vi "Word_Set_Bullet_Numbering.vi"(0 "Word._Document":refnum<k7>, 5 "start at":i32, 7 "range start":i32, 9 "range end":i32, 11 "error in (no error)":errorcluster, 12 "list index":i32, 13 "list type":i32(ring)=1 items=["wdBulletGallery"=1, "wdNumberGallery"=2, "wdOutlineNumberGallery"=3]) -> (15 "error out":errorcluster)   [LabVIEW 2017, in "NI_ReportGenerationToolkit.lvlib"]
uses:
  <vilib>/addons/_office/NI_ReportGenerationToolkit.lvlib
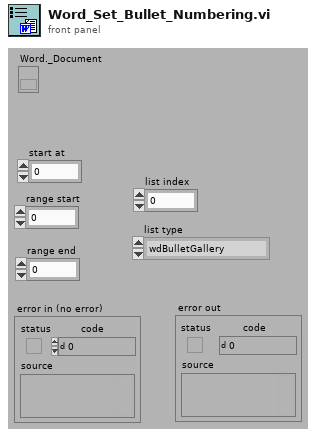
[diagram p1: front panel]
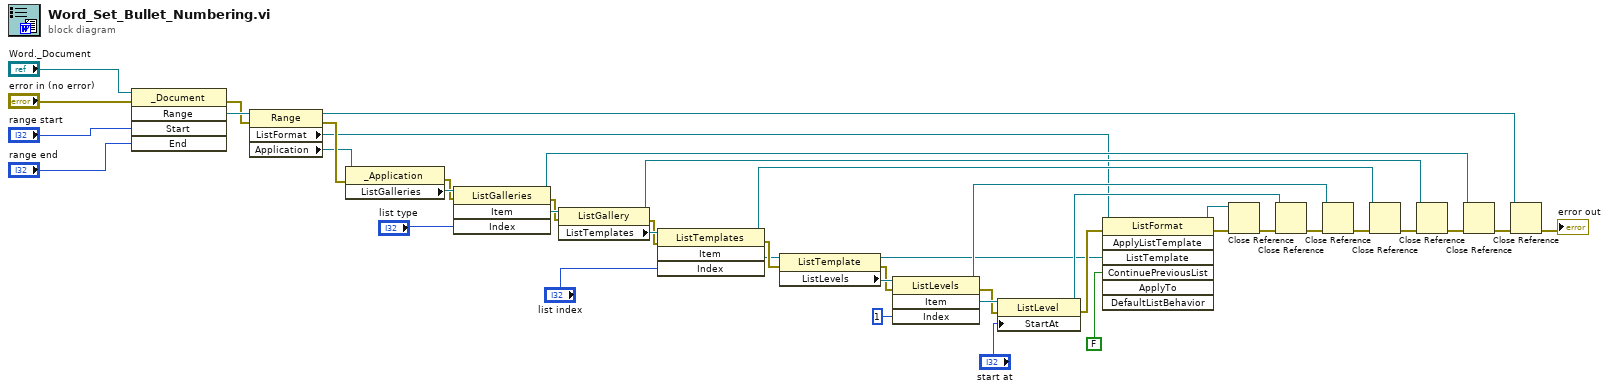
[diagram p0: block diagram]
diagram:
  n1 = invoke class="_Document" method="Range"(reference="Word._Document", error in="error in (no error)", "Start"="range start", "End"="range end") -> (error out=w26:errorcluster, "Range"=w36:refnum<k7>)  [unwired: 1 in, 3 out]
  n2 = property class="Range"(reference=w36, error in=w26) -> (reference out=w14:refnum<k7>, error out=w25:errorcluster, "ListFormat"=w4:refnum<k7>, "Application"=w7:refnum<k7>)
  n3 = property class="_Application"(reference=w7, error in=w25) -> (error out=w32:errorcluster, "ListGalleries"=w37:refnum<k7>)  [unwired: 1 out]
  n4 = invoke class="ListGalleries" method="Item"(reference=w37, error in=w32, "Index"="list type") -> (reference out=w15:refnum<k7>, error out=w31:errorcluster, "Item"=w38:refnum<k7>)  [unwired: 1 in, 1 out]
  n5 = property class="ListGallery"(reference=w38, error in=w31) -> (reference out=w18:refnum<k7>, error out=w30:errorcluster, "ListTemplates"=w39:refnum<k7>)
  n6 = invoke class="ListTemplates" method="Item"(reference=w39, error in=w30, "Index"="list index") -> (reference out=w19:refnum<k7>, error out=w29:errorcluster, "Item"=w9:refnum<k7>)  [unwired: 1 in, 1 out]
  n7 = property class="ListTemplate"(reference=w9, error in=w29) -> (reference out=w6:refnum<k7>, error out=w28:errorcluster, "ListLevels"=w40:refnum<k7>)
  n8 = invoke class="ListLevels" method="Item"(reference=w40, error in=w28, "Index"=1) -> (reference out=w11:refnum<k7>, error out=w27:errorcluster, "Item"=w41:refnum<k7>)  [unwired: 1 in, 1 out]
  n9 = property class="ListLevel"(reference=w41, error in=w27, "StartAt"="start at") -> (reference out=w10:refnum<k7>, error out=w42:errorcluster)
  n10 = invoke class="ListFormat" method="ApplyListTemplate"(reference=w4, error in=w42, "ListTemplate"=w6, "ContinuePreviousList"=FALSE) -> (reference out=w20:refnum<k7>, error out=w24:errorcluster)  [unwired: 3 in, 5 out]
  n11 = Close Reference(reference=w20, error in (no error)=w24) -> (error out=w23:errorcluster)
  n12 = Close Reference(reference=w10, error in (no error)=w23) -> (error out=w22:errorcluster)
  n13 = Close Reference(reference=w11, error in (no error)=w22) -> (error out=w5:errorcluster)
  n14 = Close Reference(reference=w19, error in (no error)=w5) -> (error out=w21:errorcluster)
  n15 = Close Reference(reference=w18, error in (no error)=w21) -> (error out=w16:errorcluster)
  n16 = Close Reference(reference=w15, error in (no error)=w16) -> (error out=w17:errorcluster)
  n17 = Close Reference(reference=w14, error in (no error)=w17) -> (error out=→"error out":errorcluster)
